vi "Celsius To Kelvin.vi"(8 "错误输入":cluster{"状态":bool, "代码":i32, "源":string}, 11 "摄氏度值":dbl) -> (0 "错误输出":cluster{"状态":bool, "代码":i32, "源":string}, 3 "绝对温度值":dbl)   [LabVIEW 2012]
uses:
  <vilib>/Utility/error.llb/Error Cluster From Error Code.vi
  <vilib>/ErrorRing/Error Ring.xnode
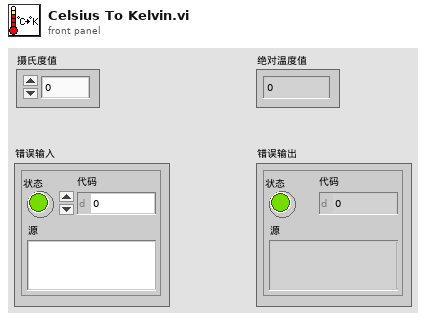
[diagram p1: front panel]
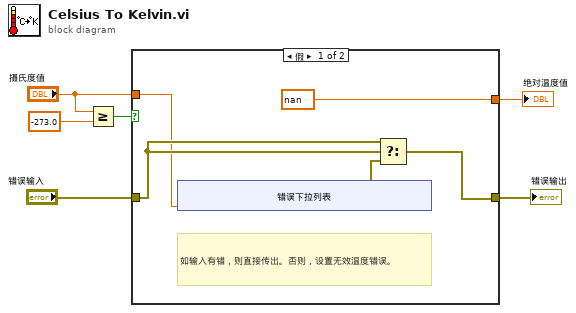
[diagram p0: block diagram]
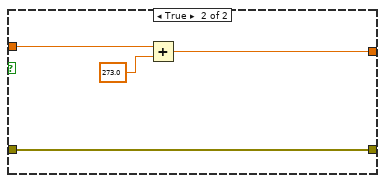
[diagram p2: hidden frame]
diagram:
  n1 = Greater Or Equal? ("大于等于？")(x="摄氏度值", y=-273.0) -> (x >= y?=w3:bool)
  n2 = case shown="假" w3 {
    tunnel: "摄氏度值" -> [w7 w22]
    tunnel: [nan w21] -> w6
    tunnel: [w9 w19] -> w2
    tunnel: "错误输入" -> [w10 w19]
    frame False {
      # "如输入有错，则直接传出。否则，设置无效温度错误。"
      n3 = xnode "错误下拉列表"("参数 0"=w7) -> ("错误输出"=w8:errorcluster)
      n4 = Select ("选择")(t=w10, s=w10, f=w8) -> (s? t:f=w9:errorcluster)
    }
    frame True {
      n5 = Add ("加")(x=w22, y=273.0) -> (x+y=w21:dbl)
    }
  }
  "绝对温度值" <- w6
  "错误输出" <- w2
